vi "Configure Generator.vi"(6 "noise level":dbl, 7 "sample rate":dbl=1000.0, 8 "error in":errorcluster, 9 "frequency":dbl=10.0, 10 "amplitude":dbl=1.0, 11 "signal type":enum32{"Sine", "Square", "Chirp"}(ring)) -> (0 "error out":errorcluster, 3 "generator settings":T1={"Amplitude"=1.0, "Frequency"=10.0, "Sample Rate"=1000.0, "Noise Level"=0.0, "Signal Type"=enum."Sine", "Block Size"=100, "Update Interval ms"=100})   [LabVIEW 2026, in "Signal Generator.lvlib"]
doc: "Configuration stage. Sanitises the user-supplied generator settings so the signal engine never receives an invalid value: amplitude and noise level are made non-negative, sample rate is coerced to 1 S/s .. 10 MS/s and frequency to 0 .. Nyquist. It also derives the streaming block size (about 100 ms of data, 16 .. 100000 samples) and the update interval in milliseconds."
uses:
  Signal Generator.lvlib
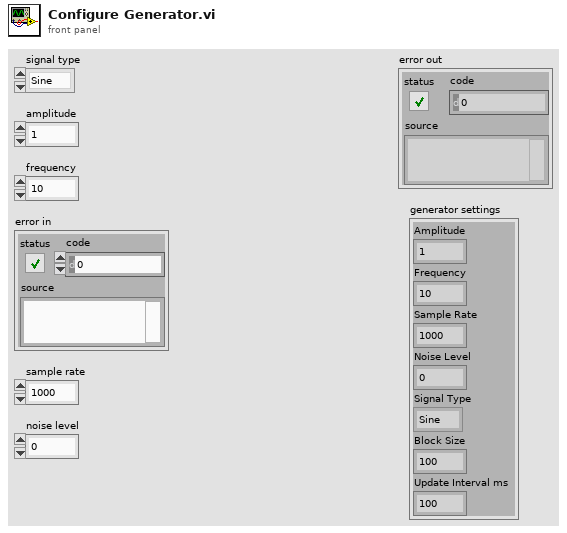
[diagram p1: front panel]
types:
  T1 = cluster{"Amplitude":dbl, "Frequency":dbl, "Sample Rate":dbl, "Noise Level":dbl, "Signal Type":enum32{"Sine", "Square", "Chirp"}, "Block Size":i32, "Update Interval ms":i32}
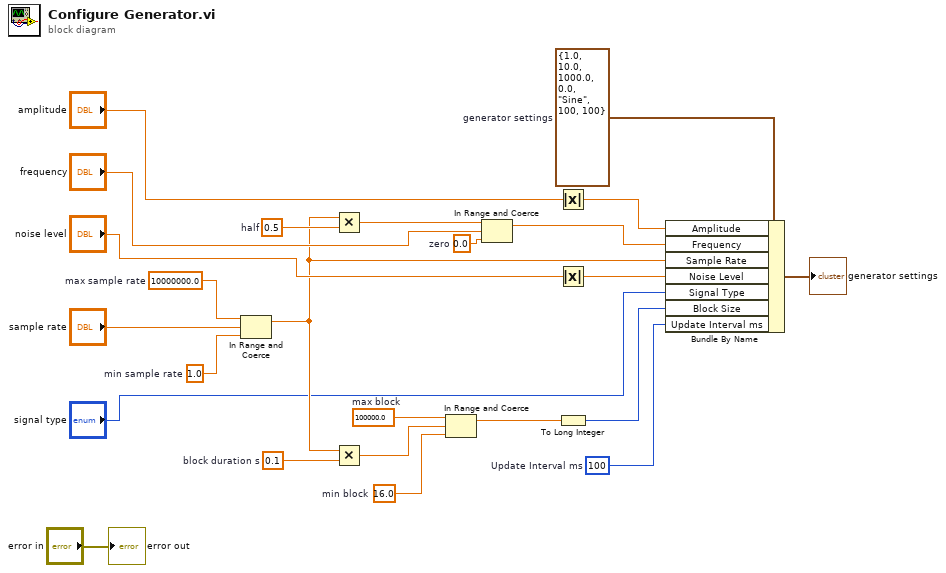
[diagram p0: block diagram]
diagram:
  w3 = T1 {"Amplitude"=1.0, "Frequency"=10.0, "Sample Rate"=1000.0, "Noise Level"=0.0, "Signal Type"=enum."Sine", "Block Size"=100, "Update Interval ms"=100}  # generator settings
  w4 = 100  # Update Interval ms
  w12 = 16.0  # min block
  w14 = 100000.0  # max block
  w15 = 0.1  # block duration s
  w16 = 0.0  # zero
  w19 = 0.5  # half
  w20 = 1.0  # min sample rate
  w22 = 10000000.0  # max sample rate
  n1 = In Range and Coerce(upper limit=w22, x="sample rate", lower limit=w20) -> (coerced(x)=w8:dbl)  [unwired: 1 out]
  n2 = Multiply(x=w8, y=w19) -> (x*y=w18:dbl)
  n3 = Multiply(x=w8, y=w15) -> (x*y=w13:dbl)
  n4 = In Range and Coerce(upper limit=w14, x=w13, lower limit=w12) -> (coerced(x)=w11:dbl)  [unwired: 1 out]
  n5 = In Range and Coerce(upper limit=w18, x="frequency", lower limit=w16) -> (coerced(x)=w9:dbl)  [unwired: 1 out]
  n6 = Absolute Value(x="amplitude") -> (abs(x)=w10:dbl)
  n7 = Absolute Value(x="noise level") -> (abs(x)=w7:dbl)
  n8 = To Long Integer(number=w11) -> (32bit integer=w5:i32)
  n9 = Bundle By Name(cluster=w3, "Amplitude"=w10, "Frequency"=w9, "Sample Rate"=w8, "Noise Level"=w7, "Signal Type"="signal type", "Block Size"=w5, "Update Interval ms"=w4) -> (→"generator settings":T1)
  "error out" <- "error in"
